vi "Open.vi"(8 "error in (no error)":errorcluster, 11 "NI Digital in":refnum<class "String Out.lvclass">) -> (0 "error out":errorcluster, 3 "NI Digital out":refnum<class "String Out.lvclass">)   [LabVIEW 2018, in "String Out.lvclass"]
doc: "String Out.lvclass:Open.vi\n\nThis is the Open VI for the String Out class. \n\nInstrument Communication Module Version 1.0\nOctober, 2020 Original Code Consulting Davita Bird\n www.originalcode.com"
uses:
  String Out.lvclass
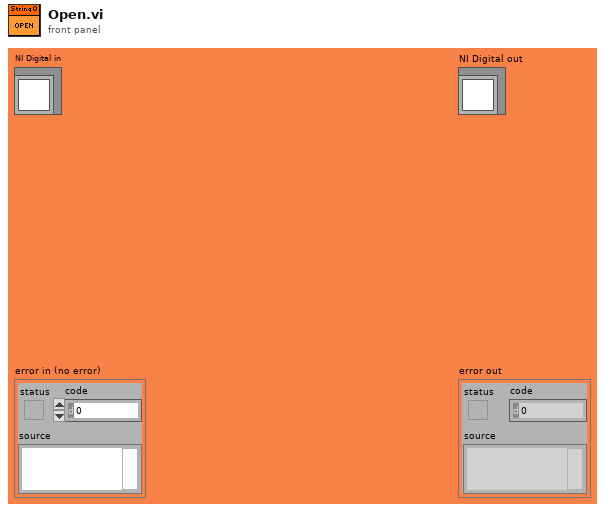
[diagram p1: front panel]
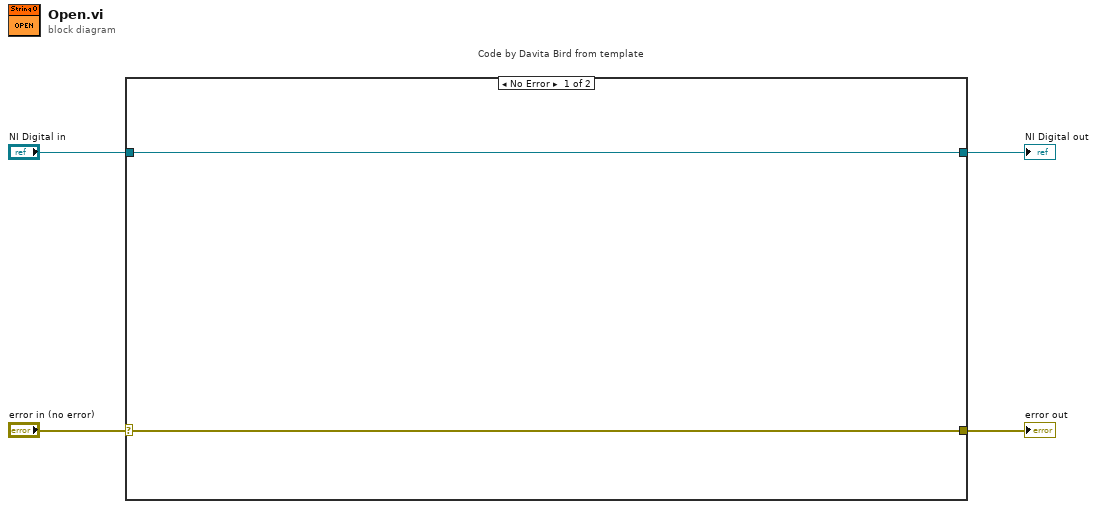
[diagram p0: block diagram]
diagram:
  n1 = case "Code by Davita Bird from template" shown="No Error" "error in (no error)" {
    selector: "error in (no error)" -> [w5 w8]
    tunnel: [w5 w8] -> w3
    tunnel: [w6 w7] -> w2
    tunnel: "NI Digital in" -> [w6 w7]
    frame No Error {
    }
    frame Error {
    }
  }
  "error out" <- w3
  "NI Digital out" <- w2
